vi "MCB2400 LED PrjAttrValidator.vi"(5 "Ctl Refnum":refnum<vi>, 9 "LEDNum (0-4)":u32(ring) items=["0", "1", "2", "3", "4", "5", "6", "7"], 11 "Attributes":T1 {"Programmable Pin Connections" items=["LED4 and Button4 use the same pin P2.10. You cannot use LED4 and Button4 in the same project.", "LED0-3 and Button0-3 use pins P0.27 and P0.28.  You cannot use LED0-3, Buton0-3, P0.27, or P0.28 in the same project."]}) -> (3 "Valid?":bool)   [LabVIEW 2011]
uses:
  <vilib>/Embedded/ARM/MCB2400/MCB2400_LED_PrjAttr.ctl
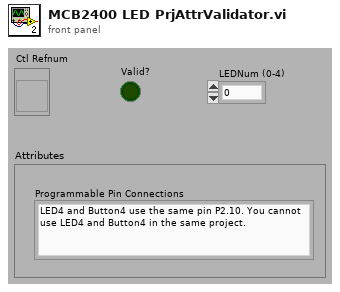
[diagram p1: front panel]
types:
  T1 = typedef "MCB2400_LED_PrjAttr.ctl" = cluster{"Programmable Pin Connections":u16}
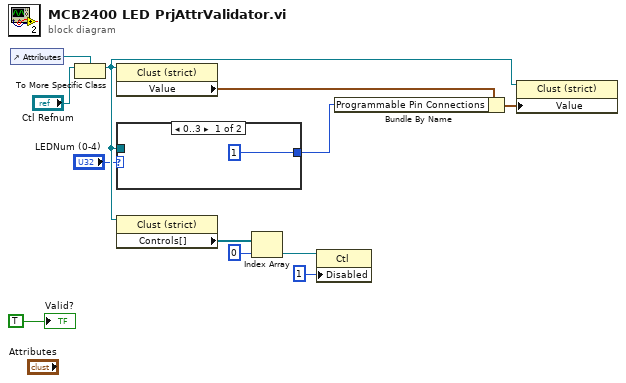
[diagram p0: block diagram]
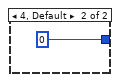
[diagram p2: hidden frame]
diagram:
  n1 = control-ref of="Attributes"() -> (w2:refnum<vi>)
  n2 = To More Specific Class(target class=w2, reference="Ctl Refnum") -> (specific class reference=w4:refnum<vi>)  [unwired: 1 in, 1 out]
  n3 = property class="Clust (strict)"(reference=w4) -> ("Value"=w11:cluster{"Programmable Pin Connections":u16})  [unwired: 1 in, 2 out]
  n4 = case shown="0..3" "LEDNum (0-4)" {
    tunnel: [u32 1 u32 0] -> w5
    tunnel: w4 -> [_ _]
    frame 0..3 {
    }
    frame 4, Default {
    }
  }
  n5 = property class="Clust (strict)"(reference=w4) -> ("Controls[]"=w9:refnum<vi>[])  [unwired: 1 in, 2 out]
  n6 = Index Array(array=w9, index=0) -> (element=w7:refnum<vi>)
  n7 = property class="Ctl"(reference=w7, "Disabled"=u8 1) -> ()  [unwired: 1 in, 2 out]
  n8 = Bundle By Name(cluster=w11, "Programmable Pin Connections"=w5) -> (w10:cluster{"Programmable Pin Connections":u16})
  n9 = property class="Clust (strict)"(reference=w4, "Value"=w10) -> ()  [unwired: 1 in, 2 out]
  "Valid?" <- TRUE ("Valid?")
